vi "about.vi"(8 "服务器信息":T1={"host"="27.154.58.30", "user"="fb", "password"="std23506", "远端地址"="/微站/室外总磷总氮高压过滤无主板新电路板/一体化微型水质监测站.exe"}, 9 "SN输入":string="SN", 10 "站点名称输入":string="站点名称", 11 "应用程序名称输入":string="地表水水质自动监测系统") -> ()   [LabVIEW 2016, in "update.lvlib"]
uses:
  update.lvlib
  <vilib>/Utility/miscctls.llb/LVPointTypeDef.ctl
panel:
  in  "检查更新":bool
  in  "更新日志":bool
  out "SN":string="SN"
  out "站点名称":string="站点名称"
  out "Version":string="Version 1.0.0"
  out "应用程序名称":string="地表水水质自动监测系统"
  # "关于"
  # "Copyright (c) 2019. All rights reserved."
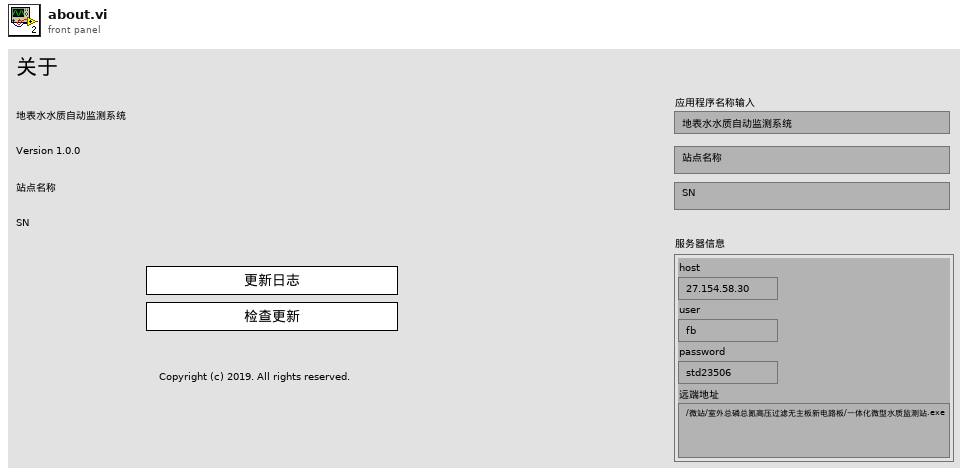
[diagram p1: front panel]
types:
  T1 = cluster{"host":string, "user":string, "password":string, "远端地址":string}
  T2 = typedef "LVPointTypeDef.ctl" = cluster{"Horizontal":i16, "Vertical":i16}
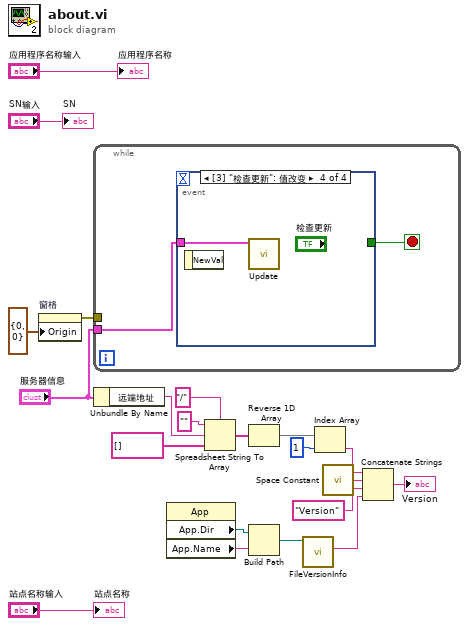
[diagram p0: block diagram]
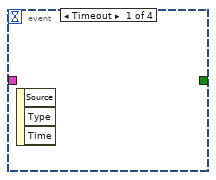
[diagram p2: hidden frame]
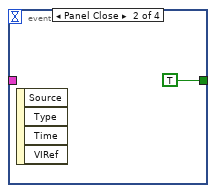
[diagram p3: hidden frame]
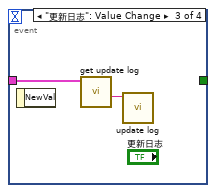
[diagram p4: hidden frame]
diagram:
  n1 = property on="窗格" class="Pane"("Origin"=T2 {"Horizontal"=0, "Vertical"=0} ("原点")) -> (error out=w20:errorcluster)  [unwired: 2 in, 1 out]
  n2 = while {
    tunnel: w20 -> [_]
    tunnel: "服务器信息" -> [w22]
    stop <- w23 stop-if-true
    n3 = event shown="[3] \"检查更新\": 值改变" {
      selector: _ -> [_ _ _ _]
      dyn-events: _ -> [_ _ _ _]
      timeout: _ -> [_ _ _ _]
      tunnel: [_ TRUE _ _] -> w23
      tunnel: w22 -> [_ _ w26 w27]
      event Timeout {
        n4 = event-data() -> ()  [unwired: 1 in, 3 out]
      }
      event Panel Close {
        n5 = event-data() -> ()  [unwired: 1 in, 4 out]
      }
      event "更新日志": Value Change {
        n6 = event-data() -> ()  [unwired: 1 in, 1 out]
        n7 = call "get update log.vi"("服务器信息"=w26) -> ("部分更新日志"=w25:string)  [unwired: 7 in, 3 out]
        n8 = call "update log.vi"("更新记录"=w25) -> ()  [unwired: 11 in]
      }
      event "检查更新": Value Change {
        n9 = event-data() -> ()  [unwired: 1 in, 1 out]
        n10 = call "Update.vi"("服务器信息"=w27) -> ()  [unwired: 11 in]
      }
    }
  }
  n11 = Unbundle By Name("服务器信息") -> ("远端地址"=w11:string)
  n12 = property class="App"() -> ("App.Dir"=w18:path, "App.Name"=w17:string)  [unwired: 2 in, 2 out]
  n13 = Spreadsheet String To Array(delimiter (Tab)="/" ("分隔符(Tab)"), format string="" ("格式字符串"), spreadsheet string=w11, array type (2D Dbl)=string[] []) -> (array=w6:string[])
  n14 = Reverse 1D Array(array=w6) -> (reversed array=w5:string[])
  n15 = Build Path(base path=w18, name or relative path=w17) -> (appended path=w16:path)
  n16 = call <vilib>:"FileVersionInfo.vi"("Application Path in"=w16) -> ("File Version Info"=w15:string)  [unwired: 7 in, 3 out]
  n17 = Index Array(array=w5, index=1 ("索引")) -> (element=w4:string)
  n18 = call <vilib>:"Space Constant.vi"() -> ("String"=w3:string)
  n19 = Concatenate Strings(w4, w3, "Version" ("字符串"), w15) -> (→"Version":string)
  "应用程序名称" <- "应用程序名称输入"
  "站点名称" <- "站点名称输入"
  "SN" <- "SN输入"
